vi "rethinkdb_tcp_query.vi"(6 "timeout ms (10000)":i32=10000, 8 "error in (no error)":errorcluster, 10 "data in":string, 11 "rethinkdb in":refnum<k5>) -> (0 "error out":errorcluster, 2 "remaining messages":string[](array[string]), 3 "rethinkdb out":refnum<k5>)   [LabVIEW 2017]
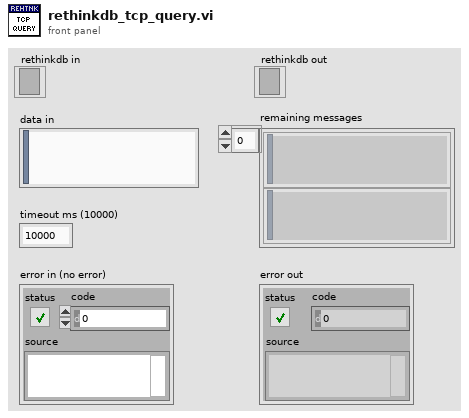
[diagram p1: front panel]
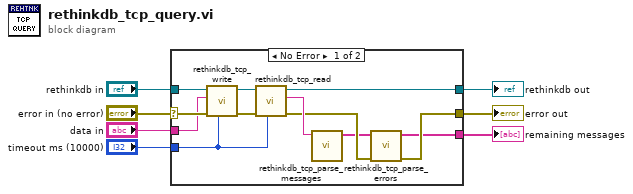
[diagram p0: block diagram]
diagram:
  n1 = case shown="No Error" "error in (no error)" {
    selector: "error in (no error)" -> [w17 w21]
    tunnel: "rethinkdb in" -> [w16 w20]
    tunnel: [w15 w20] -> w5
    tunnel: "data in" -> [w14 _]
    tunnel: "timeout ms (10000)" -> [w13 _]
    tunnel: [w10 w21] -> w2
    tunnel: [w8 _] -> w1
    frame No Error {
      n2 = call "rethinkdb_tcp_write.vi"("timeout ms (10000)"=w13, "error in (no error)"=w17, "data in"=w14, "rethinkdb in"=w16) -> ("error out"=w19:errorcluster, "rethinkdb out"=w18:refnum<k5>)  [unwired: 5 in, 1 out]
      n3 = call "rethinkdb_tcp_read.vi"("timeout ms (10000)"=w13, "error in (no error)"=w19, "rethinkdb in"=w18) -> ("error out"=w11:errorcluster, "data out"=w12:string, "rethinkdb out"=w15:refnum<k5>)  [unwired: 6 in]
      n4 = call "rethinkdb_tcp_parse_messages.vi"("data in"=w12) -> ("messages"=w9:string[])  [unwired: 9 in, 1 out]
      n5 = call "rethinkdb_tcp_parse_errors.vi"("error in (no error)"=w11, "messages"=w9) -> ("error out"=w10:errorcluster, "remaining messages"=w8:string[])  [unwired: 8 in]
    }
    frame Error {
    }
  }
  "error out" <- w2
  "rethinkdb out" <- w5
  "remaining messages" <- w1
